vi "iRobot Song Define.vi"(8 "error in":errorcluster, 9 "Notes":T2[](array[typedef]), 10 "Song Number (0-15)":u8, 11 "UART port in":T1) -> (0 "error out":errorcluster, 3 "UART port out":T1)   [LabVIEW 2010]
doc: "Define a song. Each song is alloted 16 notes, but a song can \"spill over\" into the next if so desired. The maximum number of notes that may be defined is (16 - SongNumber) * 16.\n\nThis VI writes to, but does not read from, the serial port."
uses:
  Actuator Controls/iRobot Song Note.ctl
  UART/UART Port Type.ctl
  Open Interface Controls/iRobot OpCode.ctl
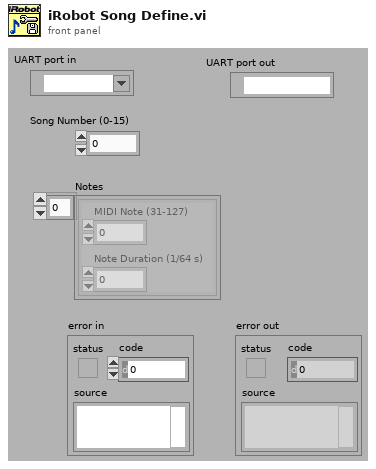
[diagram p1: front panel]
types:
  T1 = typedef "UART Port Type.ctl" = refnum<visa-resource-name>
  T2 = typedef "iRobot Song Note.ctl" = cluster{"MIDI Note (31-127)":u8, "Note Duration (1/64 s)":u8}
  T3 = typedef "iRobot OpCode.ctl" = u8
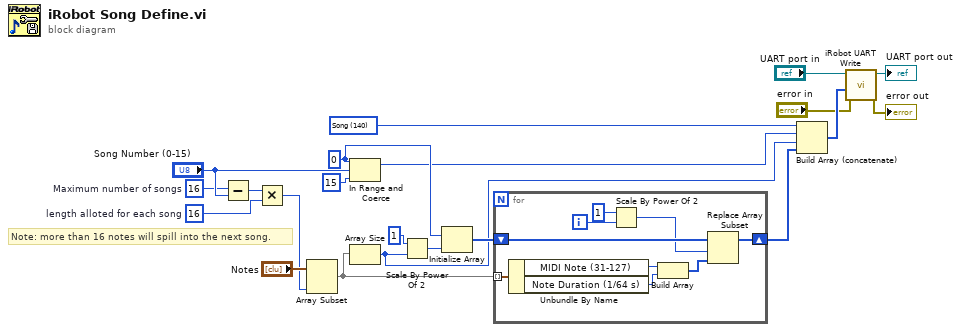
[diagram p0: block diagram]
diagram:
  w6 = u8 16  # Maximum number of songs
  w4 = 16  # length alloted for each song
  w14 = u8 0 ("upper limit")
  w15 = T3 140 items=["Start"=128, "Baud"=129, "Control"=130, "Safe"=131, "Full"=132, "Demo"=136, "Demo - Cover"=135, "Demo - Cover and Dock"=143, "Demo - Spot"=134, "Drive"=137, "Drive Direct"=145, "LEDs"=139, "Digital Outputs"=147, "PWM Low Side Drivers"=144, "Low Side Drivers"=138, "Send IR"=151, "Song"=140, "Play Song"=141, "Sensors"=142, "Query List"=149, "Stream"=148, "Pause/Resume Stream"=150, "Script"=152, "Play Script"=153, "Show Script"=154, "Wait Time"=155, "Wait Distance"=156, "Wait Angle"=157, "Wait Event"=158] ("OpCode")
  # "Note: more than 16 notes will spill into the next song."
  n1 = Subtract(x=w6, y="Song Number (0-15)") -> (x-y=w5:u8)
  n2 = Multiply(x=w5, y=w4) -> (x*y=w3:i32)
  n3 = Array Subset(array="Notes", length=w3) -> (w16:T2[])  [unwired: 1 in]
  n4 = In Range and Coerce(upper limit=w14, x="Song Number (0-15)", lower limit=u8 15) -> (coerced(x)=w13:u8)  [unwired: 1 out]
  n5 = Array Size(array=w16) -> (size(s)=w8:i32)
  n6 = Scale By Power Of 2(n=1, x=w8) -> (x*2^n=w20:i32)
  n7 = Initialize Array(w14, w20) -> (w18:u8[])
  n8 = for {
    tunnel: w16 -> [w30] mode=indexing
    shift-right: [w28] -> w9
    shift-left: w18 -> [w29]
    i -> [w27]
    n9 = Unbundle By Name(w30) -> ("MIDI Note (31-127)"=w24:u8, "Note Duration (1/64 s)"=w23:u8)
    n10 = Scale By Power Of 2(n=1, x=w27) -> (x*2^n=w25:i32)
    n11 = Build Array(w24, w23) -> (w22:u8[])
    n12 = Replace Array Subset(array=w29, new element=w22, index=w25) -> (w28:u8[])
  }
  n13 = Build Array (concatenate)(w15, w13, w8, w9) -> (w10:i32[])
  n14 = call "iRobot UART Write.vi"("error in"="error in", "data"=w10, "UART port in"="UART port in") -> ("error out"=→"error out":errorcluster, "UART port out"=→"UART port out":T1)  [unwired: 7 in]
